vi "Set Time.vi"(8 "error in (no error)":errorcluster, 10 "Set Time":cluster{"Hour":i32, "Minute":i32, "Second":i32} {"Second" min=0 max=59 step=1; "Hour" min=0 max=24 step=1; "Minute" min=0 max=59 step=1}, 11 "ARS-0220 in":refnum<class "ARS-0220.lvclass">) -> (0 "error out":errorcluster, 3 "ARS-0220 out":refnum<class "ARS-0220.lvclass">)   [LabVIEW 2021, in "Environment Chamber.lvlib" / "ARS-0220.lvclass"]
uses:
  ARS-0220.lvclass
  ARS-0220.lvclass/ARS-0220.ctl
  Support Libraries/Climatic Chamber/Climatic Chamber.lvlib
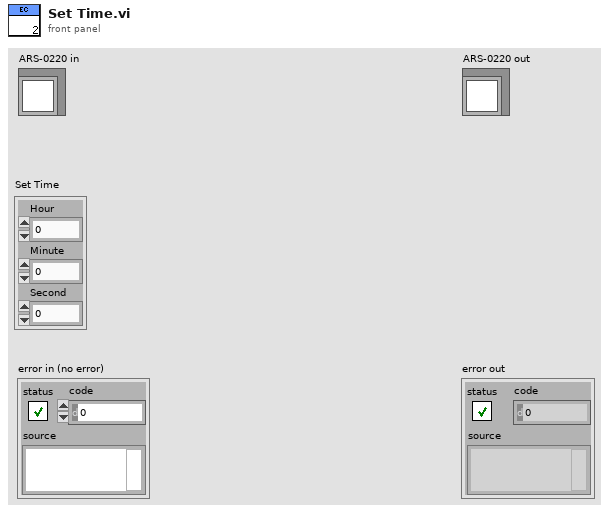
[diagram p1: front panel]
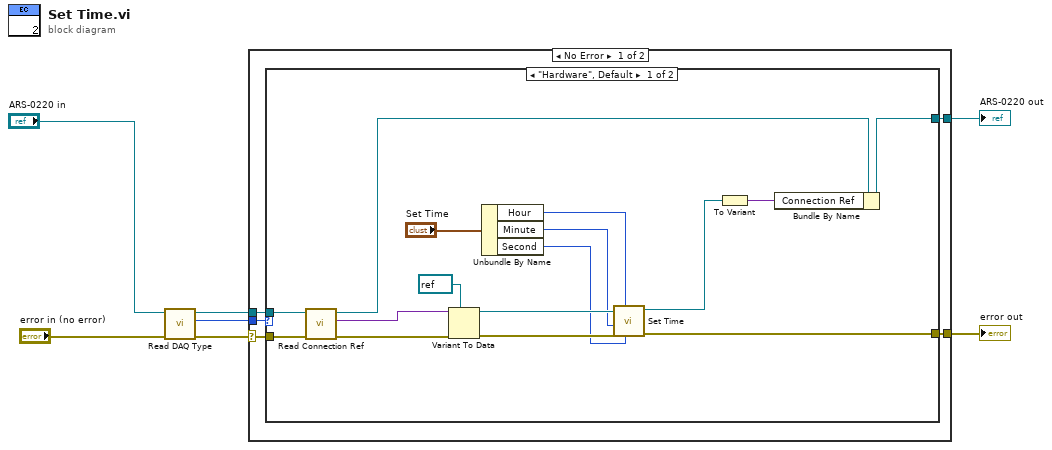
[diagram p0: block diagram]
diagram:
  n1 = call "Read DAQ Type.vi"("error in (no error)"="error in (no error)", "ARS-0220 in"="ARS-0220 in") -> ("error out"=w6:errorcluster, "DAQ Type"=w4:enum16{"Hardware", "Simulation"}, "ARS-0220 out"=w3:refnum<class "ARS-0220.lvclass">)  [unwired: 7 in]
  n2 = case shown="No Error" w6 {
    selector: w6 -> [w12 w31]
    tunnel: w4 -> [w11 _]
    tunnel: w3 -> [w10 w32]
    tunnel: [w9 w32] -> w2
    tunnel: [w8 w31] -> w1
    frame No Error {
      n3 = case shown="\"Hardware\", Default" w11 {
        tunnel: w12 -> [w28 w29]
        tunnel: w10 -> [w27 w30]
        tunnel: [w20 w30] -> w9
        tunnel: [w17 w29] -> w8
        frame "Hardware", Default {
          n4 = call "Read Connection Ref.vi"("error in (no error)"=w28, "ARS-0220 in"=w27) -> ("error out"=w26:errorcluster, "Connection Ref"=w25:variant, "ARS-0220 out"=w24:refnum<class "ARS-0220.lvclass">)  [unwired: 7 in]
          n5 = Variant To Data(error in=w26, type=refnum<visa-resource-name> refnum ("VISA resource name"), Variant=w25) -> (data=w21:refnum<visa-resource-name>, error out=w23:errorcluster)
          n6 = Unbundle By Name("Set Time") -> ("Hour"=w15:i32, "Minute"=w14:i32, "Second"=w13:i32)
          n7 = call "Set Time.vi"("Second"=w13, "Hour"=w15, "error in (no error)"=w23, "Minute"=w14, "VISA resource name"=w21) -> ("error out"=w17:errorcluster, "VISA resource name out"=w18:refnum<visa-resource-name>)  [unwired: 5 in]
          n8 = To Variant(anything=w18) -> (Variant=w19:variant)
          n9 = Bundle By Name(cluster=w24, "Connection Ref"=w19) -> (w20:refnum<class "ARS-0220.lvclass">)
        }
        frame "Simulation" {
        }
      }
    }
    frame Error {
    }
  }
  "error out" <- w1
  "ARS-0220 out" <- w2
